vi "Clear Display.vi"(6 "chip select  (1st chip)":enum16{"1st chip", "2nd chip"}(ring), 8 "error in (no error)":errorcluster, 11 "HD44780 in":refnum<class "HD44780.lvclass">) -> (0 "error out":errorcluster, 3 "HD44780 out":refnum<class "HD44780.lvclass">)   [LabVIEW 2017, in "HD44780.lvclass"]
uses:
  HD44780.lvclass
  HD44780.lvclass/HD44780.ctl
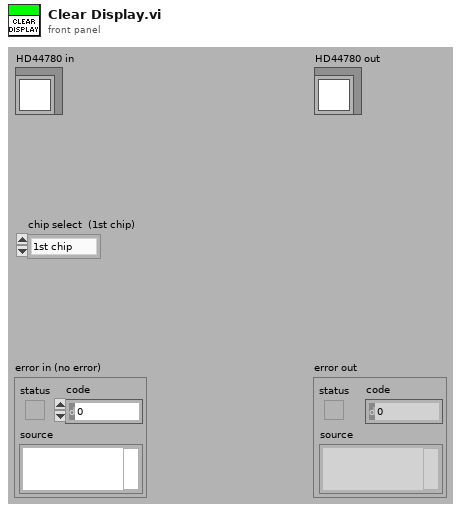
[diagram p1: front panel]
types:
  T1 = enum8{"increment & no shift", "increment & shift", "decrement & no shift", "decrement & shift"}
  T2 = typedef "HD44780 Common.lvlib/cluster of class private data.ctl" = cluster{"FPGA VI Reference":refnum<k20>, "device index":i8, "screen size":T3, "font size":T4, "auto wrap":bool, "alignment":T5, "number of line":T6, "shift 0":i8, "entry mode 0":T7, "shift 1":i8, "entry mode 1":T7}
  T3 = typedef "HD44780 Common.lvlib/screen size.ctl" = enum8{"8x1", "8x2", "12x4", "16x1", "16x2", "16x4", "20x1", "20x2", "20x4", "24x1", "24x2", "40x2", "40x4"}
  T4 = typedef "HD44780 Common.lvlib/font size.ctl" = enum8{"5x8", "5x10"}
  T5 = typedef "HD44780 Common.lvlib/alignment.ctl" = enum16{"None", "Left", "Center", "Right"}
  T6 = typedef "HD44780 Common.lvlib/line number.ctl" = enum8{"1 line", "2 lines"}
  T7 = typedef "HD44780 Common.lvlib/entry mode.ctl" = enum8{"increment & no shift", "increment & shift", "decrement & no shift", "decrement & shift"}
  T8 = cluster{"FPGA VI Reference":refnum<k20>, "device index":i8, "screen size":enum8{"8x1", "8x2", "12x4", "16x1", "16x2", "16x4", "20x1", "20x2", "20x4", "24x1", "24x2", "40x2", "40x4"}, "font size":enum8{"5x8", "5x10"}, "auto wrap":bool, "alignment":enum16{"None", "Left", "Center", "Right"}, "number of line":enum8{"1 line", "2 lines"}, "shift 0":i8, "entry mode 0":enum8{"increment & no shift", "increment & shift", "decrement & no shift", "decrement & shift"}, "shift 1":i8, "entry mode 1":enum8{"increment & no shift", "increment & shift", "decrement & no shift", "decrement & shift"}}
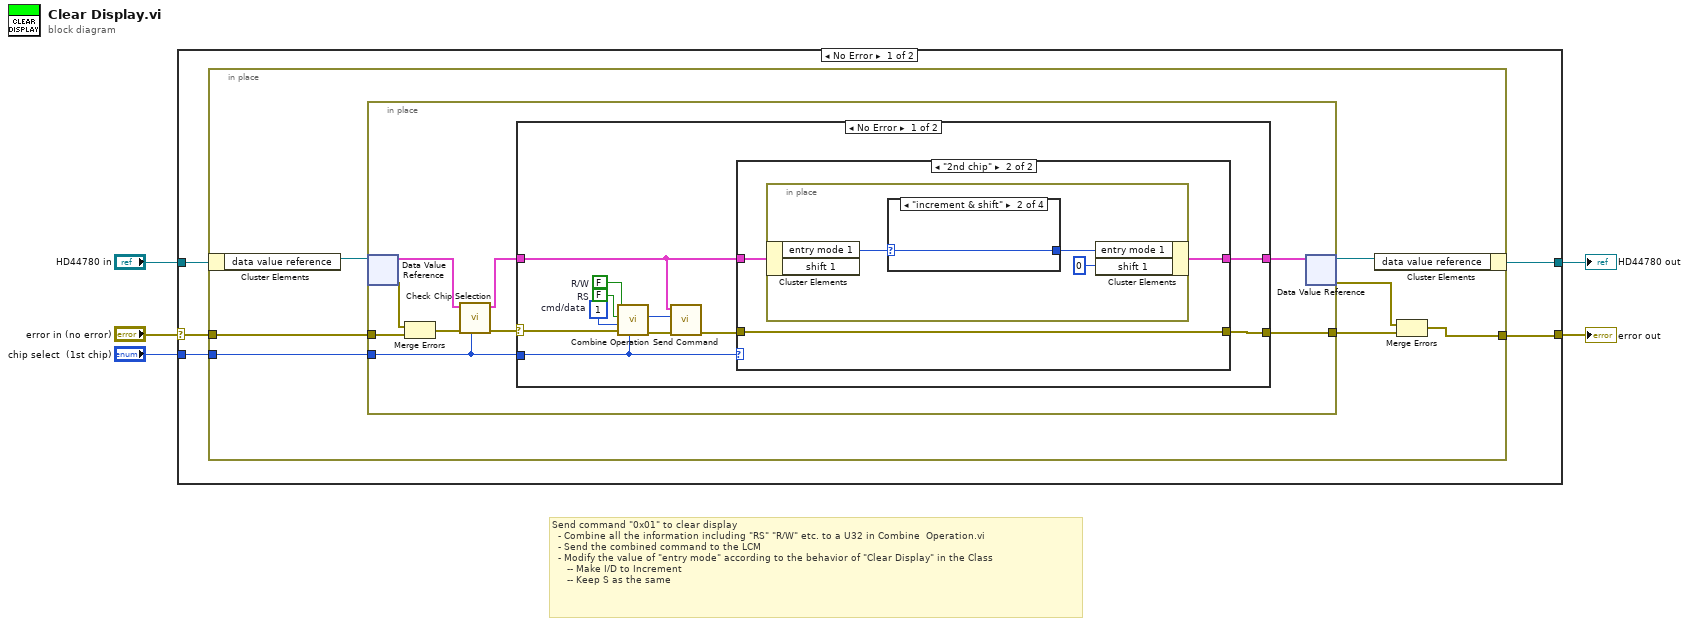
[diagram p0: block diagram]
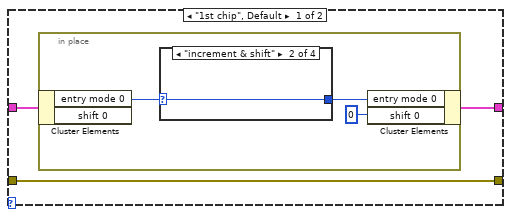
[diagram p2: hidden frame]
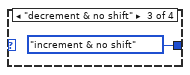
[diagram p4: hidden frame]
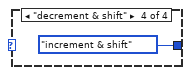
[diagram p5: hidden frame]
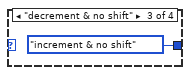
[diagram p7: hidden frame]
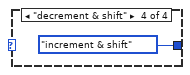
[diagram p8: hidden frame]
diagram:
  # "Send command \"0x01\" to clear display\n  - Combine all the information including \"RS\" \"R/W\" etc. to a U32 in Combine  Operation.vi \n  - Send the combined command to the LCM\n  - Modify the value of \"entry mode\" according to the behavior of \"Clear Display\" in the Class\n     -- Make I/D to Increment\n     -- Keep S as the same"
  n1 = case shown="No Error" "error in (no error)" {
    selector: "error in (no error)" -> [w6 w60]
    tunnel: "chip select  (1st chip)" -> [w10 _]
    tunnel: "HD44780 in" -> [w9 w61]
    tunnel: [w7 w60] -> w3
    tunnel: [w8 w61] -> w2
    frame No Error {
      n2 = in-place {
        in-place-border: w10 -> [w17]
        in-place-border: [w12] -> w7
        in-place-border: w6 -> [w11]
        n3 = in-place-cluster #1(w9) -> ("data value reference"=w16:refnum<data-value>)
        n4 = in-place {
          in-place-border: w17 -> [w18]
          in-place-border: [w25] -> w13
          in-place-border: w11 -> [w23]
          n5 = in-place-dvr #2(w16) -> (w19:T2, w24:errorcluster)
          n6 = Merge Errors(w24, w23) -> (w22:errorcluster)
          n7 = call "Check Chip Selection.vi"("chip select"=w18, "error in (no error)"=w22, "cluster of private data in"=w19) -> ("error out"=w21:errorcluster, "cluster of private data out"=w20:T8)  [unwired: 7 in]
          n8 = case shown="No Error" w21 {
            selector: w21 -> [w28 w58]
            tunnel: w18 -> [w27 _]
            tunnel: w20 -> [w29 w59]
            tunnel: [w34 w59] -> w26
            tunnel: [w31 w58] -> w25
            frame No Error {
              w30 = FALSE  # RS
              w36 = FALSE  # R/W
              w37 = u8 1  # cmd/data
              n9 = call "Combine Operation.vi"("chip select  (1st chip)"=w27, "error in (no error)"=w28, "cmd/data"=w37, "RS"=w30, "R/W"=w36) -> ("error out"=w35:errorcluster, "output"=w33:u32)  [unwired: 5 in]
              n10 = call "Send Command.vi"("error in (no error)"=w35, "operation"=w33, "cluster of private data in"=w29) -> ("error out"=w32:errorcluster)  [unwired: 6 in, 2 out]
              n11 = case shown="\"2nd chip\"" w27 {
                tunnel: [w40 w50] -> w34
                tunnel: w29 -> [w39 w49]
                tunnel: w32 -> [w38 w48]
                tunnel: [w38 w48] -> w31
                frame "1st chip", Default {
                  n12 = in-place {
                    n13 = in-place-cluster #3(w39) -> ("entry mode 0"=w43:T1)  [unwired: 1 out]
                    n14 = case shown="\"increment & shift\"" w43 {
                      selector: w43 -> [w44 w45 _ _]
                      tunnel: [w44 w45 T1."increment & no shift" ("entry mode 1") T1."increment & shift" ("entry mode 1")] -> w42
                      frame "increment & no shift", Default {
                      }
                      frame "increment & shift" {
                      }
                      frame "decrement & no shift" {
                      }
                      frame "decrement & shift" {
                      }
                    }
                    n15 = in-place-cluster #3("entry mode 0"=w42, "shift 0"=i8 0 ("shift 1")) -> (w40:T8)
                  }
                }
                frame "2nd chip" {
                  n16 = in-place {
                    n17 = in-place-cluster #4(w49) -> ("entry mode 1"=w53:T1)  [unwired: 1 out]
                    n18 = case shown="\"increment & shift\"" w53 {
                      selector: w53 -> [w54 w55 _ _]
                      tunnel: [w54 w55 T1."increment & no shift" ("entry mode 1") T1."increment & shift" ("entry mode 1")] -> w52
                      frame "increment & no shift", Default {
                      }
                      frame "increment & shift" {
                      }
                      frame "decrement & no shift" {
                      }
                      frame "decrement & shift" {
                      }
                    }
                    n19 = in-place-cluster #4("entry mode 1"=w52, "shift 1"=i8 0) -> (w50:T8)
                  }
                }
              }
            }
            frame Error {
            }
          }
          n20 = in-place-dvr #2(w26) -> (w15:refnum<data-value>, w14:errorcluster)
        }
        n21 = in-place-cluster #1("data value reference"=w15) -> (w8:refnum<class "HD44780.lvclass">)
        n22 = Merge Errors(w14, w13) -> (w12:errorcluster)
      }
    }
    frame Error {
    }
  }
  "error out" <- w3
  "HD44780 out" <- w2
